vi "AlliGator Get Profile Plot Name.vi"(10 "I-weighted (F)/A=weighted":bool, 11 "ratio(T)/<tau>(F)":bool) -> (3 "Plot Name Suffix":string)   [LabVIEW 2021, in "AlliGator Image Profile Window.lvlib"]
doc: "Builds plo suffix depending on user-selected options."
uses:
  AlliGator Image Profile Window.lvlib
panel:
  # "see the AlliGator License on the block diagram (Ctrl+E or Window:Show Block Diagram)"
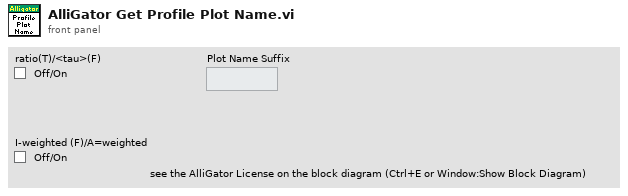
[diagram p1: front panel]
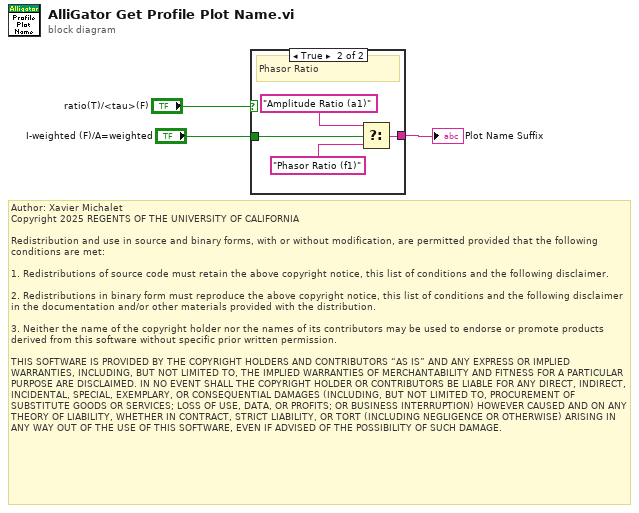
[diagram p0: block diagram]
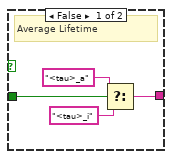
[diagram p2: hidden frame]
diagram:
  # "Author: Xavier Michalet\nCopyright 2025 REGENTS OF THE UNIVERSITY OF CALIFORNIA\n\nRedistribution and use in source and binary forms, with or without modification, are permitted provided that the following conditions are met:\n\n1. Redistributions of source code must retain the above copyright notice, this list of conditions and the following disclaimer.\n\n2. Redistributions in binary form must reproduce the above copyright notice, this list of conditions and the following disclaimer in the documentation and/or other materials provided with the distribution.\n\n3. Neither the name of the copyright holder nor the names of its contributors may be used to endorse or promote products derived from this software without specific prior written permission.\n\nTHIS SOFTWARE IS PROVIDED BY THE COPYRIGHT HOLDERS AND CONTRIBUTORS “AS IS” AND ANY EXPRESS OR IMPLIED WARRANTIES, INCLUDING, BUT NOT LIMITED TO, THE IMPLIED WARRANTIES OF MERCHANTABILITY AND FITNESS FOR A PARTICULAR PURPOSE ARE DISCLAIMED. IN NO EVENT SHALL THE COPYRIGHT HOLDER OR CONTRIBUTORS BE LIABLE FOR ANY DIRECT, INDIRECT, INCIDENTAL, SPECIAL, EXEMPLARY, OR CONSEQUENTIAL DAMAGES (INCLUDING, BUT NOT LIMITED TO, PROCUREMENT OF SUBSTITUTE GOODS OR SERVICES; LOSS OF USE, DATA, OR PROFITS; OR BUSINESS INTERRUPTION) HOWEVER CAUSED AND ON ANY THEORY OF LIABILITY, WHETHER IN CONTRACT, STRICT LIABILITY, OR TORT (INCLUDING NEGLIGENCE OR OTHERWISE) ARISING IN ANY WAY OUT OF THE USE OF THIS SOFTWARE, EVEN IF ADVISED OF THE POSSIBILITY OF SUCH DAMAGE."
  n1 = case shown="True" "ratio(T)/<tau>(F)" {
    tunnel: "I-weighted (F)/A=weighted" -> [w7 w11]
    tunnel: [w4 w10] -> w3
    frame False {
      # "Average Lifetime"
      n2 = Select(t="<tau>_a" ("Plot Name Suffix"), s=w7, f="<tau>_i" ("Plot Name Suffix")) -> (s? t:f=w4:string)
    }
    frame True {
      # "Phasor Ratio"
      n3 = Select(t="Amplitude Ratio (a1)" ("Plot Name Suffix"), s=w11, f="Phasor Ratio (f1)" ("Plot Name Suffix")) -> (s? t:f=w10:string)
    }
  }
  "Plot Name Suffix" <- w3
